vi "00 - Signal and Engineering Data Structures.vi"() -> ()   [LabVIEW 2021]
uses:
  <vilib>/Waveform/DWDTOps.llb/DWDT Search for Digital Pattern.vi
panel:
  out "normalized waveform":waveform(dbl)
  out "digital waveform out":digitalwaveform(waveform)={"t0"=timestamp(0 s since 1904-01-01), "dt"=0.0, "Y"={"transitions"=[], "data"=[]}, "error"={"status"=FALSE, "code"=37421928, "source"=""}}
  in  "integer":i32
  out "fixed-point":fxp<+,1,1> format="%.21g"
  out "r * e^(i*theta)":cdb[](array[numeric])
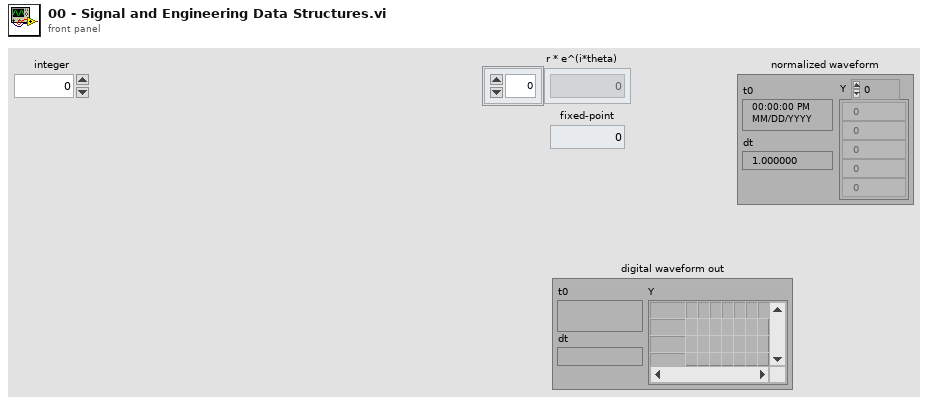
[diagram p1: front panel]
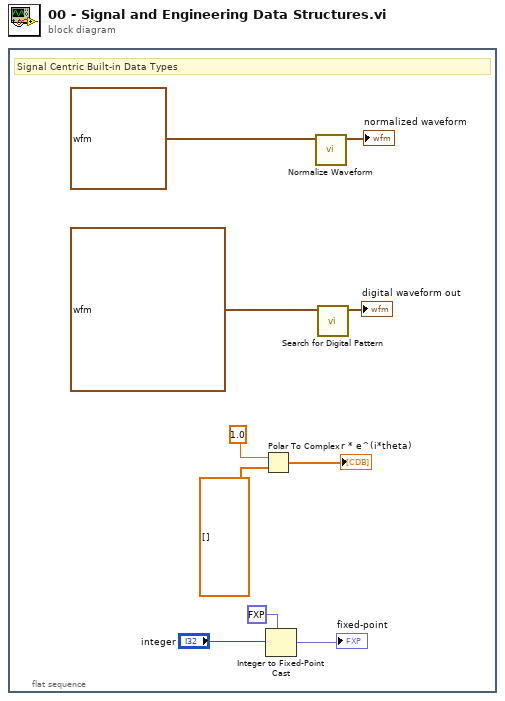
[diagram p0: block diagram]
diagram:
  n1 = flat-sequence {
    frame #0 {
      # "Signal Centric Built-in Data Types"
      n2 = Polar To Complex(1:dbl[] [] ("theta"), 2:1.0 ("r")) -> (0:→"r * e^(i*theta)":cdb[])
      n3 = Integer to Fixed-Point Cast(fixed-point type=fxp<+,1,1> 0.0, integer="integer") -> (fixed-point=→"fixed-point":fxp<+,1,1>)
      n4 = call <vilib>:"Normalize Waveform.vi"("waveform in"=waveform(dbl) {"t0"=timestamp(0 s since 1904-01-01), "dt"=1.0, "Y"=[]} ("Waveform")) -> ("normalized waveform"=→"normalized waveform":waveform(dbl))  [unwired: 7 in, 3 out]
      n5 = call-poly <vilib>:"Search for Digital Pattern.vi"("digital waveform in"=digitalwaveform {"t0"=timestamp(0 s since 1904-01-01), "dt"=0.0, "Y"={"transitions"=[], "data"=[]}, "error"={"status"=FALSE, "code"=37421928, "source"=""}}) -> ("digital waveform out"=→"digital waveform out":digitalwaveform)  [unwired: 8 in, 2 out]
    }
  }
